vi "Result_Test.vi"(8 "error in (no error)":errorcluster caption="entrée d'erreur (pas d'erreur)", 11 "Get_Voltage en entrée":refnum<class "Nodon_Generate_SN.lvclass">) -> (0 "error out":errorcluster caption="sortie d'erreur", 3 "Get_Voltage en sortie":refnum<class "Nodon_Generate_SN.lvclass">)   [LabVIEW 2020, in "Library Test.lvlib" / "Nodon_Generate_SN.lvclass"]
uses:
  Nodon_Generate_SN.lvclass
  C:/Users/ngarcin/OneDrive - Altyor/Standard TB/Suite TB45/Class/Test/Test (Default)/Test (Default).lvclass
  Commun VI/TypeDef/Variable Printable.ctl
  Test_Wtih_Instr/Test_With_Inst.lvclass
  Commun VI/Library Commun.lvlib
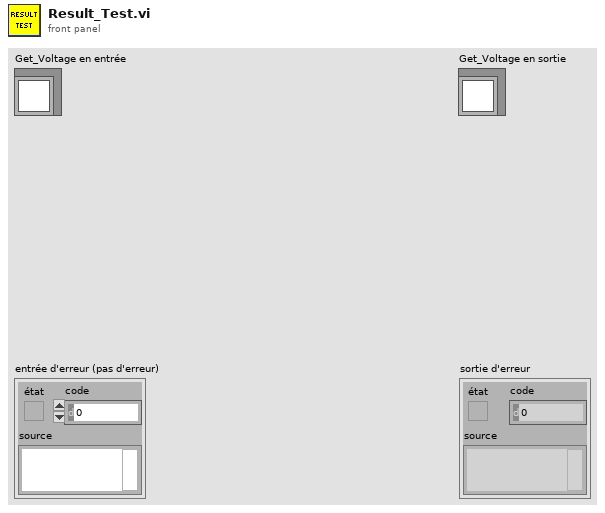
[diagram p1: front panel]
types:
  T1 = typedef "Variable Printable.ctl" = string
  T2 = enum16{"Get Variable", "Get All Variables", "Set Variable", "Delete Variable", "Delete All Variable"}
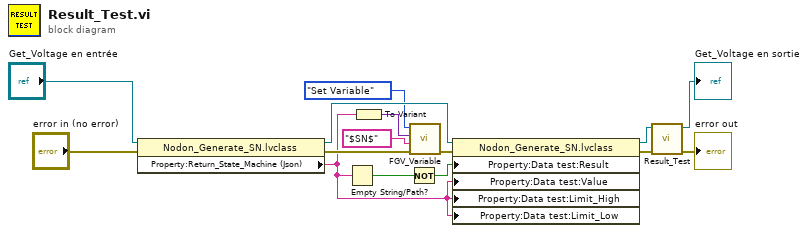
[diagram p0: block diagram]
diagram:
  n1 = property class="Nodon_Generate_SN.lvclass"(reference="Get_Voltage en entrée", error in="error in (no error)") -> (reference out=w12:refnum<class "Nodon_Generate_SN.lvclass">, error out=w6:errorcluster, "Property:Return_State_Machine (Json)"=w3:string)
  n2 = Empty String/Path?(string/path=w3) -> (empty?=w2:bool)
  n3 = To Variant(anything=w3) -> (Variant=w4:variant)
  n4 = Not(x=w2) -> (.not. x?=w1:bool)
  n5 = call "FGV_Variable.vi"("error in (no error)"=w6, "Variable"=T1 "$SN$" ("Variable Printable"), "Data In"=w4, "Function"=T2."Set Variable") -> ("error out"=w5:errorcluster)  [unwired: 5 in, 2 out]
  n6 = property class="Nodon_Generate_SN.lvclass"(reference=w12, error in=w5, "Property:Data test:Result"=w1, "Property:Data test:Value"=w3, "Property:Data test:Limit_High"=w3, "Property:Data test:Limit_Low"=w3) -> (reference out=w9:refnum<class "Nodon_Generate_SN.lvclass">, error out=w10:errorcluster)
  n7 = call-parent "Result_Test.vi"("error in (no error)"=w10, "Test_With_Inst en entrée"=w9) -> ("error out"=→"error out":errorcluster, "Test_With_Inst en sortie"=→"Get_Voltage en sortie":refnum<class "Nodon_Generate_SN.lvclass">)  [unwired: 8 in]
